vi "Logging - SET -  Actor_Name.vi"(8 "error in (no error)":errorcluster, 10 "Actor_Name IN":string, 11 "Logging_Class in":refnum<class "Logging_Class.lvclass">) -> (0 "error out":errorcluster, 2 "Actor Name Out":string, 3 "Logging_Class out":refnum<class "Logging_Class.lvclass">)   [LabVIEW 2023, in "Logging.lvlib" / "Logging_Class.lvclass"]
uses:
  Logging_Class.lvclass
  Logging_Class.lvclass/Logging_Class.ctl
  <vilib>/Utility/error.llb/Trim Whitespace One-Sided.vi
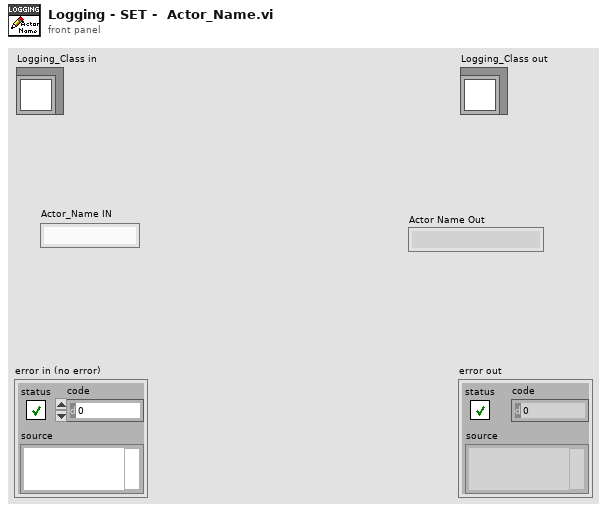
[diagram p1: front panel]
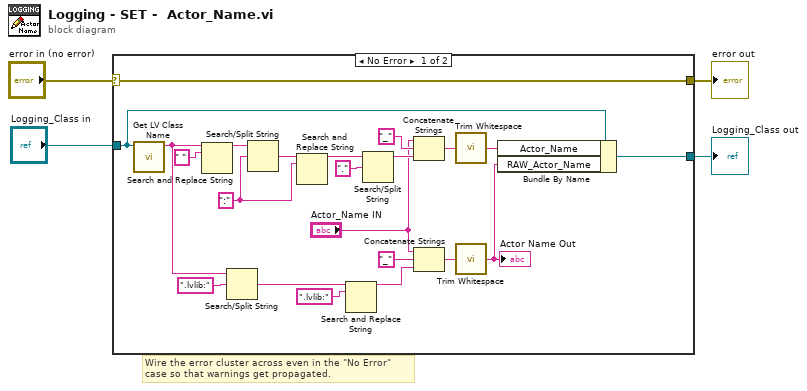
[diagram p0: block diagram]
diagram:
  # "Wire the error cluster across even in the \"No Error\"\ncase so that warnings get propagated."
  n1 = case shown="No Error" "error in (no error)" {
    selector: "error in (no error)" -> [w26 w28]
    tunnel: [w26 w28] -> w3
    tunnel: [w9 w27] -> w1
    tunnel: "Logging_Class in" -> [w7 w27]
    frame No Error {
      w22 = ":" ("search string/char (-)")
      n2 = call <vilib>:"Get LV Class Name.vi"("object"=w7) -> ("class name"=w12:string)  [unwired: 9 in, 1 out]
      n3 = Search and Replace String(input string=w12, search string=" ") -> (result string=w24:string)  [unwired: 6 in, 3 out]
      n4 = Search/Split String(string=w12, search string/char (-)=".lvlib:") -> (match + rest of string=w15:string)  [unwired: 1 in, 2 out]
      n5 = Search/Split String(string=w24, search string/char (-)=w22) -> (match + rest of string=w23:string)  [unwired: 1 in, 2 out]
      n6 = Search and Replace String(input string=w23, search string=w22) -> (result string=w19:string)  [unwired: 6 in, 3 out]
      n7 = Search and Replace String(input string=w15, search string=".lvlib:" ("search string/char (-)")) -> (result string=w14:string)  [unwired: 6 in, 3 out]
      n8 = Search/Split String(string=w19, search string/char (-)=".") -> (substring before match=w17:string)  [unwired: 1 in, 2 out]
      n9 = Concatenate Strings("Actor_Name IN", "_" ("string"), w17) -> (w20:string)
      n10 = Concatenate Strings("Actor_Name IN", "_" ("string"), w14) -> (w13:string)
      n11 = call <vilib>:"Trim Whitespace.vi"("string"=w20) -> ("trimmed string"=w8:string)  [unwired: 1 in]
      n12 = call <vilib>:"Trim Whitespace.vi"("string"=w13) -> ("trimmed string"=w6:string)  [unwired: 1 in]
      "Actor Name Out" <- w6
      n13 = Bundle By Name(cluster=w7, "Actor_Name"=w8, "RAW_Actor_Name"=w6) -> (w9:refnum<class "Logging_Class.lvclass">)
    }
    frame Error {
    }
  }
  "error out" <- w3
  "Logging_Class out" <- w1
